vi "Keithley 2400 Source Set.vi"(7 "Source Type":enum16{"Voltage Source", "Current Source"}(ring), 8 "error in (no error)":errorcluster, 10 "Voltage/curent Level":dbl, 11 "VISA Refnum in":refnum<visa-resource-name>) -> (0 "error out":errorcluster, 3 "VISA Refnum out":refnum<visa-resource-name>)   [LabVIEW 2019]
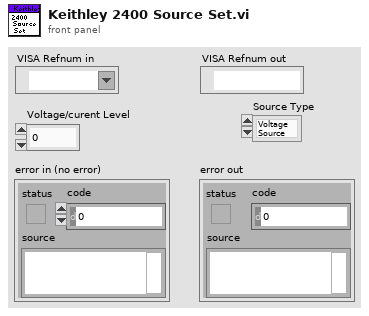
[diagram p1: front panel]
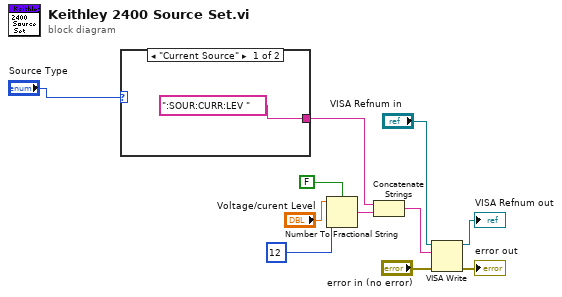
[diagram p0: block diagram]
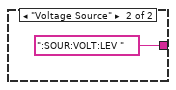
[diagram p2: hidden frame]
diagram:
  n1 = case shown="\"Current Source\"" "Source Type" {
    tunnel: [":SOUR:CURR:LEV " ":SOUR:VOLT:LEV "] -> w5
    frame "Current Source" {
    }
    frame "Voltage Source" {
    }
  }
  n2 = Number To Fractional String(use system decimal point (T)=FALSE, number="Voltage/curent Level", precision (6)=i16 12) -> (F-format string=w4:string)  [unwired: 1 in]
  n3 = Concatenate Strings(w5, w4) -> (w6:string)
  n4 = VISA Write(VISA resource name="VISA Refnum in", write buffer=w6, error in (no error)="error in (no error)") -> (VISA resource name out=→"VISA Refnum out":refnum<visa-resource-name>, error out=→"error out":errorcluster)  [unwired: 1 out]
